vi "Scripting_Server_loop.vi"(4 "error in (no error)":errorcluster, 6 "queue in":refnum<queue>, 7 "TCP Connection ID":refnum<k5>) -> (0 "error out":errorcluster, 3 "Shutdown?":bool)   [LabVIEW 2015]
uses:
  Users/Sherman/Desktop/BETA_GSCS/Systems/SystemUtil/Command.ctl
  Utils/ChangeConfig.ctl
  Utils/ChangeSI.ctl
  Utils/ChangeTCS.ctl
  Users/Sherman/Desktop/BETA_GSCS/Systems/Slit/slitactions.ctl
  TCPServer/TCP_Global.vi
panel:
  out "Focus Done":bool
  out "Focus Commanded":bool
  out "Camset Done":bool
  out "Setup Done":bool
  out "Setup Commanded":bool
  out "Config Server":bool
  out "SI Server":bool
  out "TCS Server":bool
  out "Exposure Active?":bool
  out "Command History":string
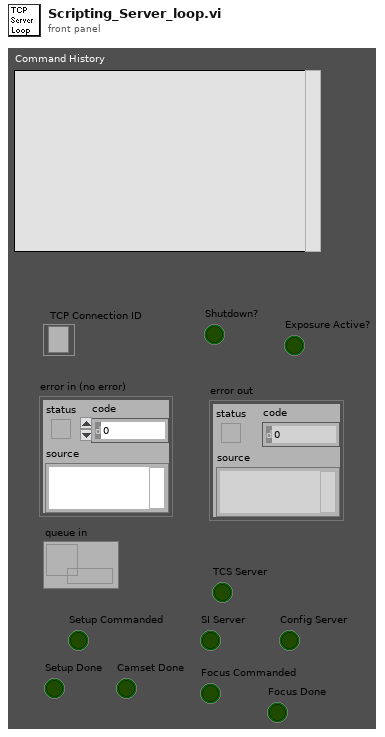
[diagram p1: front panel]
types:
  T1 = typedef "ChangeTCS.ctl" = cluster{"Command":string, "TCS":cluster{"Comp Mirror":bool, "RA":string, "DEC":string, "Epoch":string}}
  T2 = typedef "ChangeSI.ctl" = cluster{"Command":string, "SI camera info":cluster{"Observer Name":string, "object name":string, "File name base":string, "Camera Color":string, "Exp type tab":enum16{"Object", "Flat", "Comp", "Dark", "Zero", "Focus"}, "Number of Exp":i32, "Exp time":i32, "CCD Readout Speed":u8, "CCD ROI Mode":u16, "Hg(Ar)":bool, "Cu":bool, "Ne":bool, "Bulb":bool, "Ar":bool, "Quartz":bool, "Quartz Percent":i32, "Fe":bool, "Notes":string, "Target Number":string, "DomePercent":i32, "Dome":bool, "Start":dbl, "Delta":dbl, "Steps":dbl, "Custom Roi":cluster{i32, i32, i32, i32, i32, i32}}}
  T3 = typedef "ChangeConfig.ctl" = cluster{"Command":string, "Configuration":cluster{"Primary Filter":string, "Secondary Filter":string, "Slit Mask":string, "Grating":string, "CS Target":dbl, "GS Target":dbl, "Coll Focus":i32, "Camera Focus":i32, "use Flexure Comp?":bool, "WavMode":string, "Slit Toggle":string}}
  T4 = typedef "Command.ctl" = cluster{"Command":string, "Parameter":string}
  T5 = typedef "slitactions.ctl" = enum16{"Launch", "INIT_CTL", "Restart", "Show", "Hide", "Home", "Move", "Rotate Only", "Shutdown"}
  T6 = typedef "ThreadStates.ctl" = enum16{"Waiting", "Scripting", "Uninitialized", "Error"}
  T7 = cluster{"GT Thread state":T6, "Slit Thread State":T6, "F1 Thread State":T6, "F2 Thread State":T6, "Coll Thread State":T6, "CF Thread State":T6, "Wavelength Thread State":T6}
  T8 = cluster{"Grating Name":string, "Slit Name":string, "Primary Filter Name":string, "Secondary Filter name":string, "Coll Position":i32, "Camera Focus":i32, "Camera Angle":dbl, "Grating Angle":dbl, "Coll Temp":dbl, "CF Temp\n":dbl, "Camera Target":dbl, "Grating Target":dbl, "WAVMODE":string, "Slit Hidden??":bool}
  T9 = cluster{"String":string, "String":string, "String":string, "String":string, "String":string, "String":string}
  T10 = cluster{"String":dbl, "String":dbl, "String":dbl, "String":dbl, "String":dbl, "String":dbl}
  T11 = cluster{"String":string, "String":string, "String":string, "String":string, "String":string, "String":string, "String":string, "String":string}
  T12 = cluster{"String":bool, "String":bool, "String":bool, "String":bool, "String":bool, "String":bool, "String":bool, "String":bool}
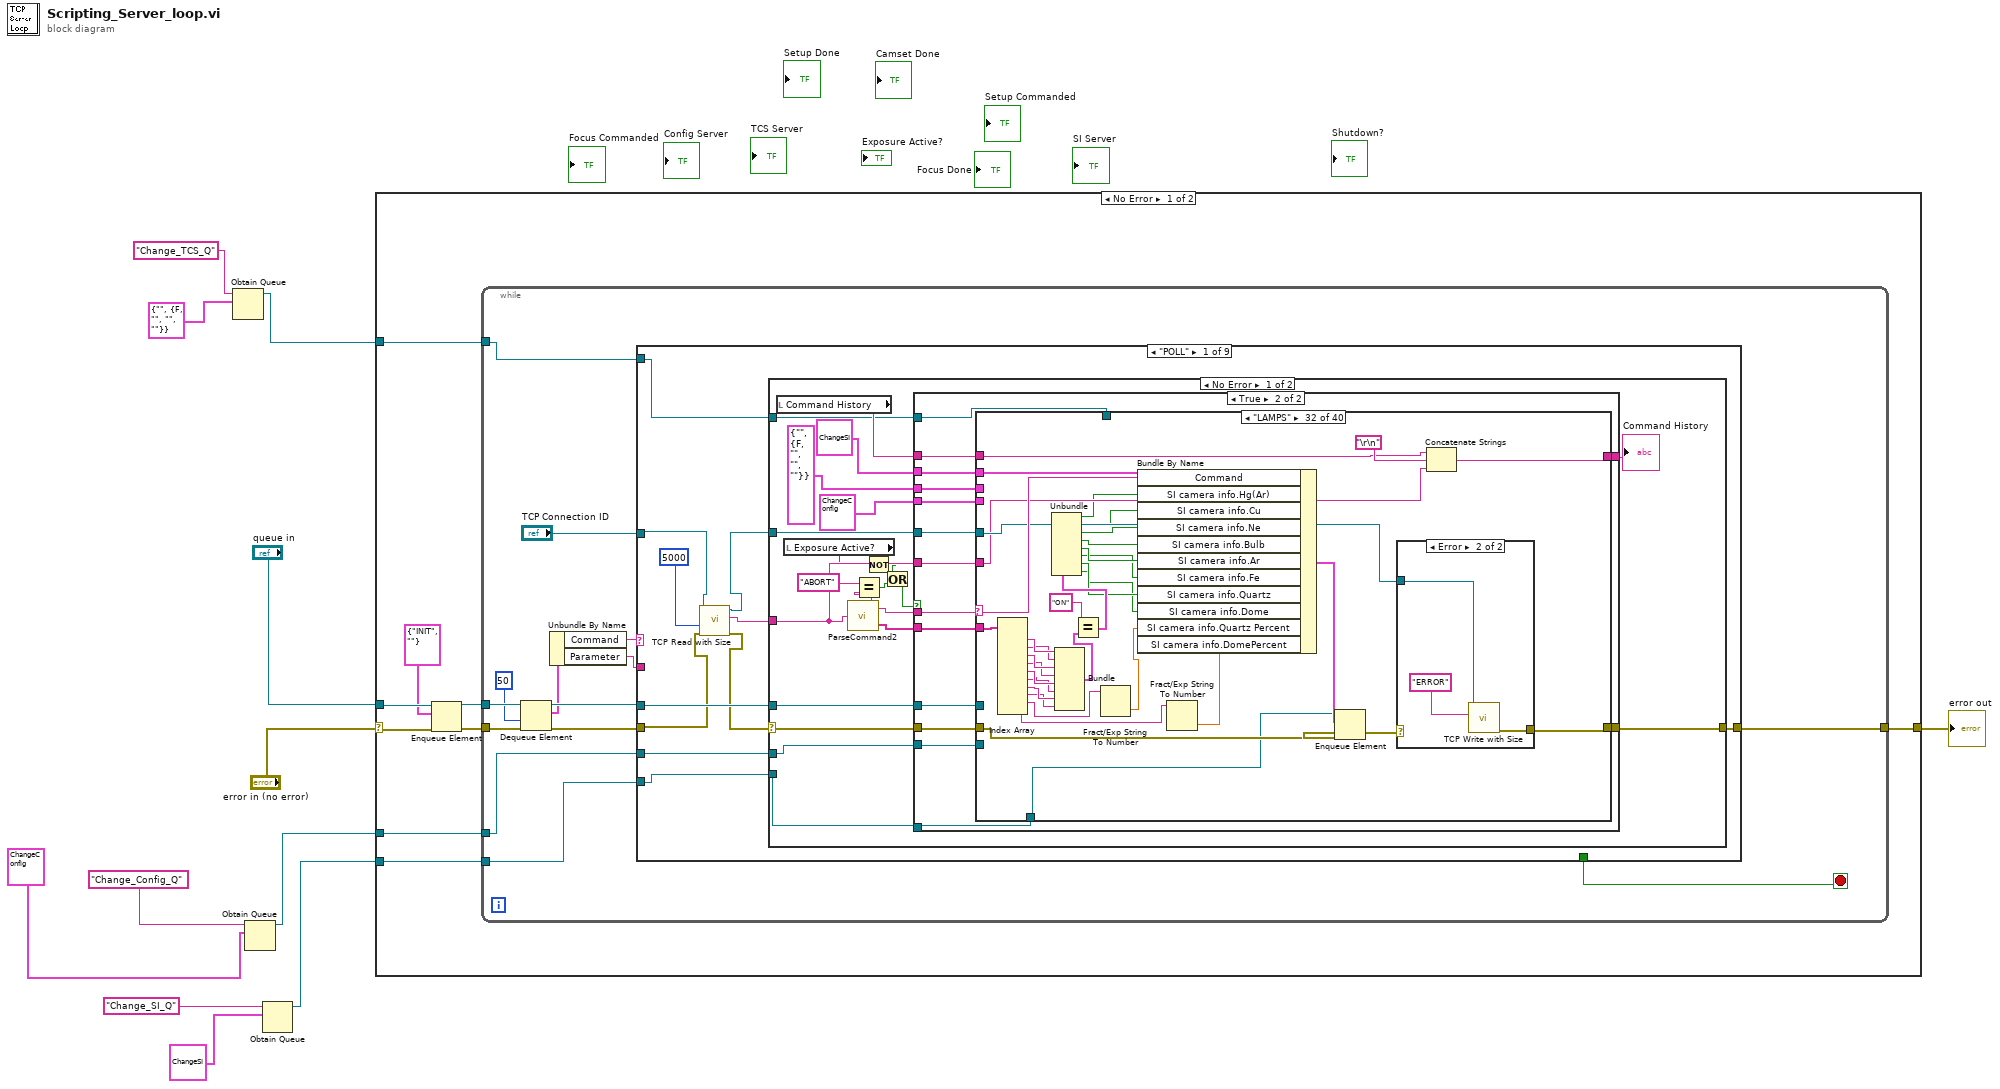
[diagram p0: block diagram]
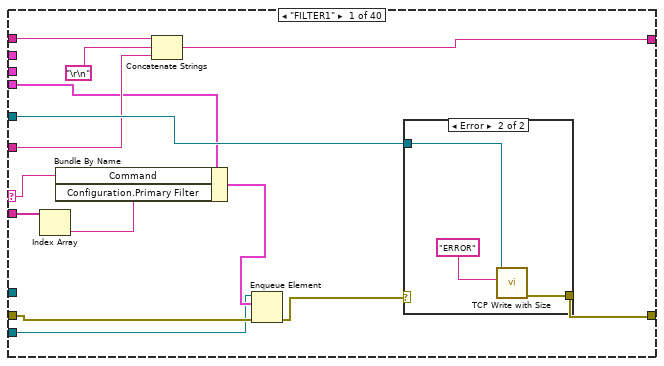
[diagram p3: hidden frame]
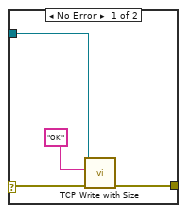
[diagram p4: hidden frame]
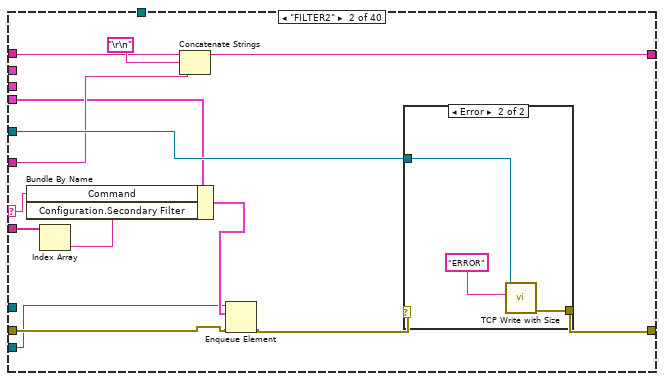
[diagram p5: hidden frame]
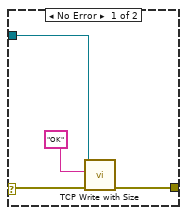
[diagram p6: hidden frame]
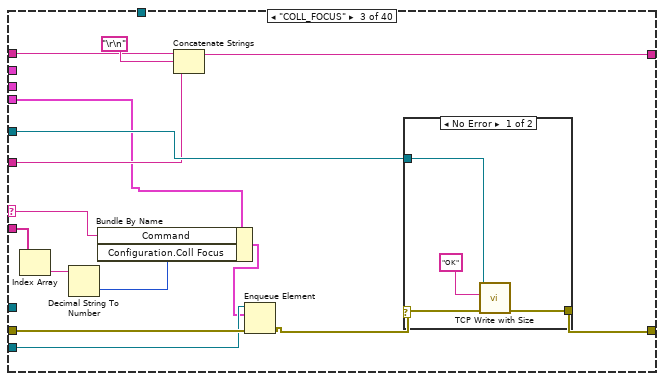
[diagram p7: hidden frame]
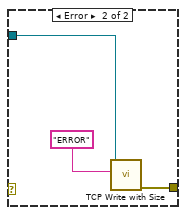
[diagram p8: hidden frame]
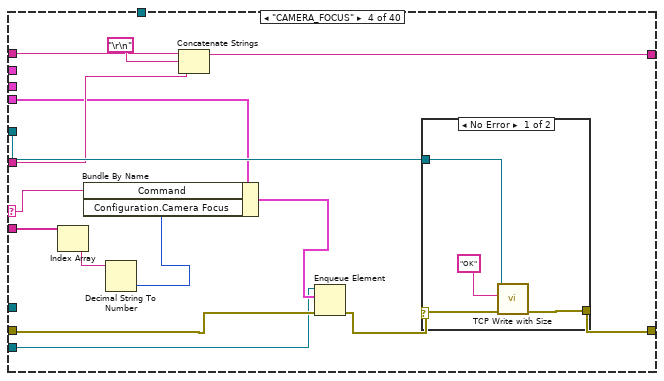
[diagram p9: hidden frame]
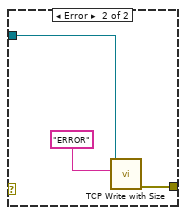
[diagram p10: hidden frame]
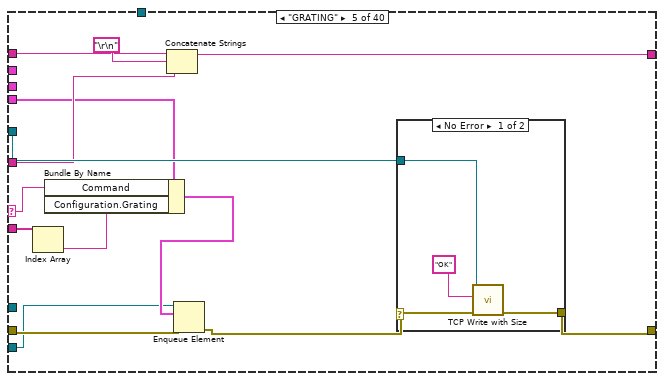
[diagram p11: hidden frame]
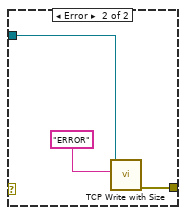
[diagram p12: hidden frame]
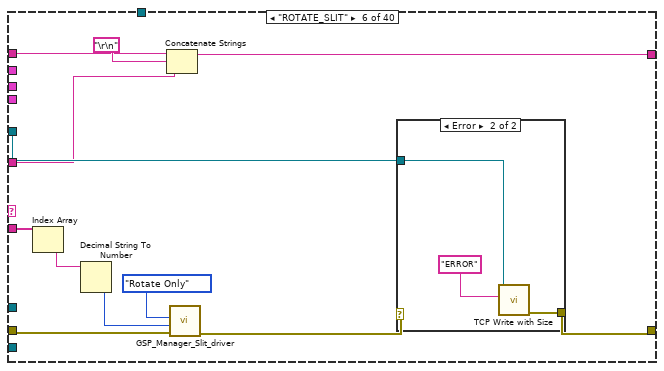
[diagram p13: hidden frame]
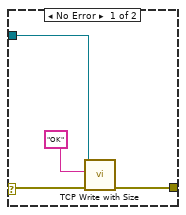
[diagram p14: hidden frame]
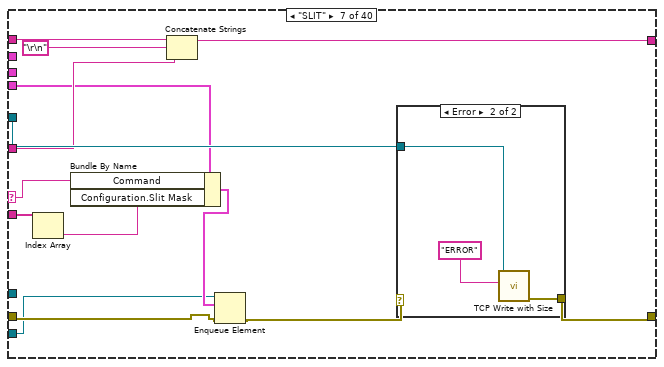
[diagram p15: hidden frame]
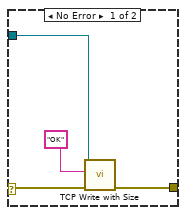
[diagram p16: hidden frame]
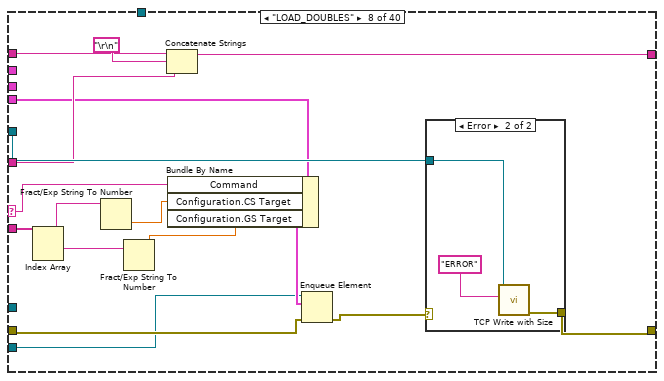
[diagram p17: hidden frame]
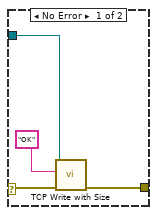
[diagram p18: hidden frame]
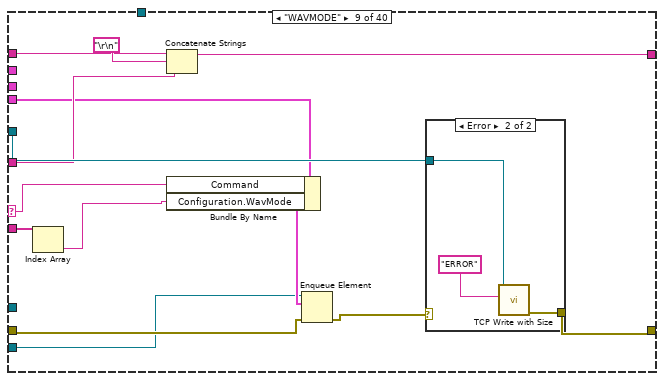
[diagram p19: hidden frame]
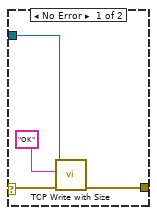
[diagram p20: hidden frame]
diagram:
  n1 = Obtain Queue(name (unnamed)="Change_TCS_Q", element data type=T1 {"Command"="", "TCS"={"Comp Mirror"=FALSE, "RA"="", "DEC"="", "Epoch"=""}} ("Cluster")) -> (queue out=w2:refnum<queue>)  [unwired: 3 in, 2 out]
  n2 = Obtain Queue(name (unnamed)="Change_Config_Q", element data type=T3 {"Command"="", "Configuration"={"Primary Filter"="", "Secondary Filter"="", "Slit Mask"="", "Grating"="", "CS Target"=0.0, "GS Target"=0.0, "Coll Focus"=0, "Camera Focus"=0, "use Flexure Comp?"=FALSE, "WavMode"="", "Slit Toggle"=""}} ("Cluster")) -> (queue out=w8:refnum<queue>)  [unwired: 3 in, 2 out]
  n3 = Obtain Queue(name (unnamed)="Change_SI_Q", element data type=T2 {"Command"="", "SI camera info"={"Observer Name"="", "object name"="", "File name base"="", "Camera Color"="Red", "Exp type tab"=enum."Object", "Number of Exp"=0, "Exp time"=0, "CCD Readout Speed"=5, "CCD ROI Mode"=10, "Hg(Ar)"=FALSE, "Cu"=FALSE, "Ne"=FALSE, "Bulb"=FALSE, "Ar"=FALSE, "Quartz"=FALSE, "Quartz Percent"=0, "Fe"=FALSE, "Notes"="", "Target Number"="", "DomePercent"=0, "Dome"=FALSE, "Start"=0.0, "Delta"=0.0, "Steps"=0.0, "Custom Roi"={0, 4096, 1, 0, 4096, 1}}} ("Cluster")) -> (queue out=w5:refnum<queue>)  [unwired: 3 in, 2 out]
  n4 = case shown="No Error" "error in (no error)" {
    selector: "error in (no error)" -> [w17 w1141]
    tunnel: [w21 w1141] -> w11
    tunnel: "queue in" -> [w18 _]
    tunnel: w8 -> [w15 _]
    tunnel: w5 -> [w14 _]
    tunnel: w2 -> [w13 _]
    frame No Error {
      n5 = Enqueue Element(queue=w18, element=T4 {"Command"="INIT", "Parameter"=""}, error in (no error)=w17) -> (queue out=w20:refnum<queue>, error out=w19:errorcluster)  [unwired: 1 in, 1 out]
      n6 = while {
        tunnel: w20 -> [w35]
        tunnel: [w31] -> w21
        tunnel: w19 -> [w30]
        tunnel: w15 -> [w26]
        tunnel: w14 -> [w25]
        tunnel: w13 -> [w23]
        stop <- w22 stop-if-true
        n7 = Dequeue Element(queue=w35, timeout in ms (-1)=50, error in (no error)=w30) -> (queue out=w33:refnum<queue>, element=w29:T4, error out=w34:errorcluster)  [unwired: 1 out]
        n8 = Unbundle By Name(w29) -> ("Command"=w28:string, "Parameter"=w24:string)
        n9 = case shown="\"POLL\"" w28 {
          tunnel: w33 -> [w45 _ _ _ w1061 _ _ _ _]
          tunnel: w34 -> [w40 w985 w1031 w1056 w1062 w1096 w1101 w1106 w1129]
          tunnel: "TCP Connection ID" -> [w42 w992 w1032 w1057 w1058 _ _ w1105 _]
          tunnel: [w46 w991 w1030 w1055 w1060 w1096 w1101 w1106 w1126] -> w31
          tunnel: [_ _ _ _ _ _ _ TRUE _] -> w22
          tunnel: w26 -> [w44 _ _ _ _ _ _ _ _]
          tunnel: w25 -> [w43 _ _ _ _ _ _ _ _]
          tunnel: w24 -> [_ w986 w1035 w1053 _ w1095 w1100 _ _]
          tunnel: w23 -> [w36 _ _ _ _ _ _ _ _]
          frame "POLL" {
            n10 = call "TCP Read with Size.vi"("error in (no error)"=w40, "timeout ms (25000)"=5000, "connection ID"=w42) -> ("error out"=w39:errorcluster, "data out"=w38:string, "connection ID out"=w37:refnum<k5>)  [unwired: 6 in]
            n11 = case shown="No Error" w39 {
              selector: w39 -> [w64 w980]
              tunnel: w38 -> [w56 _]
              tunnel: w37 -> [w66 _]
              tunnel: [w63 w979] -> w46
              tunnel: w45 -> [w65 _]
              tunnel: w44 -> [w60 _]
              tunnel: w43 -> [w59 _]
              tunnel: w36 -> [w54 _]
              frame No Error {
                n12 = local read "Command History"() -> (w62:string)
                n13 = local read "Exposure Active?"() -> (w50:bool)
                n14 = call "ParseCommand2.vi"("Command string"=w56) -> ("Command"=w51:string, "Parameters"=w55:string[])
                n15 = Equal?(x="ABORT", y=w51) -> (x = y?=w49:bool)
                n16 = Not(x=w50) -> (.not. x?=w48:bool)
                n17 = Or(x=w48, y=w49) -> (x .or. y?=w47:bool)
                n18 = case shown="True" w47 {
                  tunnel: w66 -> [_ w83]
                  tunnel: w65 -> [_ w82]
                  tunnel: w64 -> [w68 w81]
                  tunnel: [w68 w80] -> w63
                  tunnel: w62 -> [w67 w79]
                  tunnel: [w67 w78] -> w61
                  tunnel: w60 -> [_ w77]
                  tunnel: w59 -> [_ w76]
                  tunnel: T3 {"Command"="", "Configuration"={"Primary Filter"="", "Secondary Filter"="", "Slit Mask"="", "Grating"="", "CS Target"=0.0, "GS Target"=0.0, "Coll Focus"=0, "Camera Focus"=0, "use Flexure Comp?"=FALSE, "WavMode"="", "Slit Toggle"=""}} ("Cluster") -> [_ w75]
                  tunnel: T2 {"Command"="", "SI camera info"={"Observer Name"="", "object name"="", "File name base"="Red", "Camera Color"="", "Exp type tab"=enum."Object", "Number of Exp"=0, "Exp time"=0, "CCD Readout Speed"=5, "CCD ROI Mode"=10, "Hg(Ar)"=FALSE, "Cu"=FALSE, "Ne"=FALSE, "Bulb"=FALSE, "Ar"=FALSE, "Quartz"=FALSE, "Quartz Percent"=0, "Fe"=FALSE, "Notes"="", "Target Number"="", "DomePercent"=0, "Dome"=FALSE, "Start"=0.0, "Delta"=0.0, "Steps"=0.0, "Custom Roi"={0, 4096, 1, 0, 4096, 1}}} ("SI camera info") -> [_ w74]
                  tunnel: w56 -> [_ w73]
                  tunnel: w51 -> [_ w72]
                  tunnel: w55 -> [_ w71]
                  tunnel: w54 -> [_ w70]
                  tunnel: T1 {"Command"="", "TCS"={"Comp Mirror"=FALSE, "RA"="", "DEC"="", "Epoch"=""}} ("Cluster") -> [_ w69]
                  frame False {
                    # "do not accept commands other than abort when exposure is active"
                    # "exposure is active and command is not abort"
                  }
                  frame True {
                    n19 = case shown="\"LAMPS\"" w72 {
                      selector: w72 -> [w86 w107 w127 w150 w172 _ w212 w234 w258 w279 w304 _ _ _ w350 w379 w401 w425 w447 w476 w498 w519 w540 w561 w585 w603 w627 w648 w673 w697 w720 w765 w803 w831 w875 w892 w910 _ w947 _]
                      tunnel: w83 -> [w96 w117 w139 w161 w183 w199 w223 w246 w268 w289 w305 w322 w334 w345 w360 w380 w402 w420 w448 w472 w499 w520 w541 w562 w581 w601 w628 w647 w674 w696 w719 w764 w806 w832 w876 w890 w908 w934 w954 w967]
                      tunnel: w71 -> [w97 w118 w140 w159 w182 w197 w222 w245 w267 w288 w303 _ _ _ w357 w378 w400 w424 w446 w475 w497 w518 w539 _ w584 w604 w626 w649 w672 w698 w721 w766 w804 w824 w871 _ _ w925 w949 _]
                      tunnel: w82 -> [_ _ _ _ _ _ _ _ _ _ _ _ _ _ _ _ _ _ _ _ _ _ _ _ _ _ _ _ _ _ _ _ _ _ _ _ _ _ _ _]
                      tunnel: w81 -> [w89 w110 w132 w153 w175 w198 w215 w236 w260 w281 w298 w320 w335 w346 w361 w377 w399 w423 w445 w474 w494 w515 w537 w560 w582 w605 w625 w650 w671 w699 w723 w768 w801 w830 w873 _ _ _ _ w965]
                      tunnel: [w95 w116 w138 w160 w181 w196 w221 w244 w266 w287 w297 w323 w336 w347 w358 w376 w398 w419 w443 w459 w493 w514 w535 w558 w580 w596 w623 w652 w669 w688 w717 w762 w807 w833 w878 w888 w906 w933 w953 w966] -> w80
                      tunnel: w79 -> [w93 w114 w136 w157 w179 w194 w219 w242 w264 w285 w309 w324 w332 w343 w352 w372 w395 w417 w441 w470 w491 w511 w533 w554 w575 w599 w621 w644 w667 w691 w715 w760 w786 w828 w859 w897 w915 w937 w957 w970]
                      tunnel: w73 -> [w92 w112 w134 w155 w177 w192 w217 w240 w262 w283 w306 _ _ _ w349 w371 w393 w415 w440 w469 w490 w510 w532 w553 w574 w598 w620 w643 w666 w690 w714 w759 w785 w827 w858 w896 w914 w936 w956 w969]
                      tunnel: [w94 w113 w135 w156 w178 w193 w218 w241 w263 w284 w308 w324 w332 w343 w351 w373 w394 w416 w439 w468 w489 w512 w531 w552 w573 w597 w619 w642 w665 w689 w713 w758 w784 w826 w860 w895 w913 w935 w955 w968] -> w78
                      tunnel: w77 -> [w84 w105 w131 w148 w170 _ w210 w231 w256 w277 w299 _ _ _ _ _ _ _ _ _ _ _ _ _ _ _ _ _ _ _ _ _ w802 _ _ _ _ _ _ _]
                      tunnel: w76 -> [_ _ _ _ _ _ _ _ _ _ _ _ _ _ w354 w375 w397 w422 w444 w473 w495 w516 w536 w559 w583 w606 w624 w651 w670 w700 w722 w767 _ w819 w874 w891 w909 _ _ _]
                      tunnel: w75 -> [w87 w108 w126 w151 w173 _ w213 w233 w257 w278 w307 _ _ _ _ _ _ _ _ _ _ _ _ _ _ _ _ _ _ _ _ _ w805 _ _ _ _ _ _ _]
                      tunnel: w74 -> [_ _ _ _ _ _ _ _ _ _ _ _ _ _ w362 w381 w403 w421 w449 w477 w500 w521 w542 w563 w586 w602 w629 w646 w675 w695 w718 w763 _ w825 w877 w889 w907 _ _ _]
                      tunnel: w70 -> [_ _ _ _ _ _ _ _ _ _ _ _ _ _ _ _ _ _ _ _ _ _ _ _ _ _ _ _ _ _ _ _ _ _ _ _ _ w932 w952 _]
                      tunnel: w69 -> [_ _ _ _ _ _ _ _ _ _ _ _ _ _ _ _ _ _ _ _ _ _ _ _ _ _ _ _ _ _ _ _ _ _ _ _ _ w931 w951 _]
                      frame "FILTER1" {
                        n20 = Index Array(array=w97) -> (element=w85:string)  [unwired: 1 in]
                        n21 = Bundle By Name(cluster=w87, "Command"=w86, "Configuration.Primary Filter"=w85) -> (w90:T3)
                        n22 = Concatenate Strings(w93, "\r\n", w92) -> (w94:string)
                        n23 = Enqueue Element(queue=w84, element=w90, error in (no error)=w89) -> (error out=w88:errorcluster)  [unwired: 1 in, 2 out]
                        n24 = case shown="Error" w88 {
                          selector: w88 -> [w98 _]
                          tunnel: w96 -> [w100 w102]
                          tunnel: [w99 w103] -> w95
                          frame No Error {
                            n25 = call "TCP Write with Size.vi"("error in (no error)"=w98, "data in"="OK", "connection ID"=w100) -> ("error out"=w99:errorcluster)  [unwired: 6 in, 2 out]
                          }
                          frame Error {
                            n26 = call "TCP Write with Size.vi"("data in"="ERROR", "connection ID"=w102) -> ("error out"=w103:errorcluster)  [unwired: 7 in, 2 out]
                          }
                        }
                      }
                      frame "FILTER2" {
                        n27 = Index Array(array=w118) -> (element=w106:string)  [unwired: 1 in]
                        n28 = Bundle By Name(cluster=w108, "Command"=w107, "Configuration.Secondary Filter"=w106) -> (w111:T3)
                        n29 = Concatenate Strings(w114, "\r\n", w112) -> (w113:string)
                        n30 = Enqueue Element(queue=w105, element=w111, error in (no error)=w110) -> (error out=w109:errorcluster)  [unwired: 1 in, 2 out]
                        n31 = case shown="Error" w109 {
                          selector: w109 -> [w119 _]
                          tunnel: w117 -> [w121 w124]
                          tunnel: [w120 w123] -> w116
                          frame No Error {
                            n32 = call "TCP Write with Size.vi"("error in (no error)"=w119, "data in"="OK", "connection ID"=w121) -> ("error out"=w120:errorcluster)  [unwired: 6 in, 2 out]
                          }
                          frame Error {
                            n33 = call "TCP Write with Size.vi"("data in"="ERROR", "connection ID"=w124) -> ("error out"=w123:errorcluster)  [unwired: 7 in, 2 out]
                          }
                        }
                      }
                      frame "COLL_FOCUS" {
                        n34 = Index Array(array=w140) -> (element=w129:string)  [unwired: 1 in]
                        n35 = Decimal String To Number(string=w129) -> (number=w130:i32)  [unwired: 2 in, 1 out]
                        n36 = Bundle By Name(cluster=w126, "Command"=w127, "Configuration.Coll Focus"=w130) -> (w128:T3)
                        n37 = Concatenate Strings(w136, "\r\n", w134) -> (w135:string)
                        n38 = Enqueue Element(queue=w131, element=w128, error in (no error)=w132) -> (error out=w133:errorcluster)  [unwired: 1 in, 2 out]
                        n39 = case shown="No Error" w133 {
                          selector: w133 -> [w141 _]
                          tunnel: w139 -> [w143 w146]
                          tunnel: [w142 w145] -> w138
                          frame No Error {
                            n40 = call "TCP Write with Size.vi"("error in (no error)"=w141, "data in"="OK", "connection ID"=w143) -> ("error out"=w142:errorcluster)  [unwired: 6 in, 2 out]
                          }
                          frame Error {
                            n41 = call "TCP Write with Size.vi"("data in"="ERROR", "connection ID"=w146) -> ("error out"=w145:errorcluster)  [unwired: 7 in, 2 out]
                          }
                        }
                      }
                      frame "CAMERA_FOCUS" {
                        n42 = Index Array(array=w159) -> (element=w162:string)  [unwired: 1 in]
                        n43 = Decimal String To Number(string=w162) -> (number=w152:i32)  [unwired: 2 in, 1 out]
                        n44 = Bundle By Name(cluster=w151, "Command"=w150, "Configuration.Camera Focus"=w152) -> (w154:T3)
                        n45 = Concatenate Strings(w157, "\r\n", w155) -> (w156:string)
                        n46 = Enqueue Element(queue=w148, element=w154, error in (no error)=w153) -> (error out=w149:errorcluster)  [unwired: 1 in, 2 out]
                        n47 = case shown="No Error" w149 {
                          selector: w149 -> [w163 _]
                          tunnel: w161 -> [w165 w168]
                          tunnel: [w164 w167] -> w160
                          frame No Error {
                            n48 = call "TCP Write with Size.vi"("error in (no error)"=w163, "data in"="OK", "connection ID"=w165) -> ("error out"=w164:errorcluster)  [unwired: 6 in, 2 out]
                          }
                          frame Error {
                            n49 = call "TCP Write with Size.vi"("data in"="ERROR", "connection ID"=w168) -> ("error out"=w167:errorcluster)  [unwired: 7 in, 2 out]
                          }
                        }
                      }
                      frame "GRATING" {
                        n50 = Index Array(array=w182) -> (element=w171:string)  [unwired: 1 in]
                        n51 = Bundle By Name(cluster=w173, "Command"=w172, "Configuration.Grating"=w171) -> (w176:T3)
                        n52 = Concatenate Strings(w179, "\r\n", w177) -> (w178:string)
                        n53 = Enqueue Element(queue=w170, element=w176, error in (no error)=w175) -> (error out=w174:errorcluster)  [unwired: 1 in, 2 out]
                        n54 = case shown="No Error" w174 {
                          selector: w174 -> [w184 _]
                          tunnel: w183 -> [w186 w189]
                          tunnel: [w185 w188] -> w181
                          frame No Error {
                            n55 = call "TCP Write with Size.vi"("error in (no error)"=w184, "data in"="OK", "connection ID"=w186) -> ("error out"=w185:errorcluster)  [unwired: 6 in, 2 out]
                          }
                          frame Error {
                            n56 = call "TCP Write with Size.vi"("data in"="ERROR", "connection ID"=w189) -> ("error out"=w188:errorcluster)  [unwired: 7 in, 2 out]
                          }
                        }
                      }
                      frame "ROTATE_SLIT" {
                        n57 = Index Array(array=w197) -> (element=w202:string)  [unwired: 1 in]
                        n58 = Decimal String To Number(string=w202) -> (number=w201:i32)  [unwired: 2 in, 1 out]
                        n59 = Concatenate Strings(w194, "\r\n", w192) -> (w193:string)
                        n60 = call "GSP_Manager_Slit_driver.vi"("error in (no error)"=w198, "Slit # (Move/Rotate Only)"=w201, "Action"=slitactions."Rotate Only") -> ("error out"=w200:errorcluster)  [unwired: 3 in, 1 out]
                        n61 = case shown="Error" w200 {
                          selector: w200 -> [w203 _]
                          tunnel: w199 -> [w205 w208]
                          tunnel: [w204 w207] -> w196
                          frame No Error {
                            n62 = call "TCP Write with Size.vi"("error in (no error)"=w203, "data in"="OK", "connection ID"=w205) -> ("error out"=w204:errorcluster)  [unwired: 6 in, 2 out]
                          }
                          frame Error {
                            n63 = call "TCP Write with Size.vi"("data in"="ERROR", "connection ID"=w208) -> ("error out"=w207:errorcluster)  [unwired: 7 in, 2 out]
                          }
                        }
                      }
                      frame "SLIT" {
                        n64 = Index Array(array=w222) -> (element=w211:string)  [unwired: 1 in]
                        n65 = Bundle By Name(cluster=w213, "Command"=w212, "Configuration.Slit Mask"=w211) -> (w216:T3)
                        n66 = Concatenate Strings(w219, "\r\n", w217) -> (w218:string)
                        n67 = Enqueue Element(queue=w210, element=w216, error in (no error)=w215) -> (error out=w214:errorcluster)  [unwired: 1 in, 2 out]
                        n68 = case shown="Error" w214 {
                          selector: w214 -> [w224 _]
                          tunnel: w223 -> [w226 w229]
                          tunnel: [w225 w228] -> w221
                          frame No Error {
                            n69 = call "TCP Write with Size.vi"("error in (no error)"=w224, "data in"="OK", "connection ID"=w226) -> ("error out"=w225:errorcluster)  [unwired: 6 in, 2 out]
                          }
                          frame Error {
                            n70 = call "TCP Write with Size.vi"("data in"="ERROR", "connection ID"=w229) -> ("error out"=w228:errorcluster)  [unwired: 7 in, 2 out]
                          }
                        }
                      }
                      frame "LOAD_DOUBLES" {
                        n71 = Index Array(array=w245) -> (element #1=w247:string, element #2=w239:string)  [unwired: 2 in]
                        n72 = Fract/Exp String To Number(string=w247) -> (number=w232:dbl)  [unwired: 3 in, 1 out]
                        n73 = Fract/Exp String To Number(string=w239) -> (number=w237:dbl)  [unwired: 3 in, 1 out]
                        n74 = Concatenate Strings(w242, "\r\n", w240) -> (w241:string)
                        n75 = Bundle By Name(cluster=w233, "Command"=w234, "Configuration.CS Target"=w232, "Configuration.GS Target"=w237) -> (w238:T3)
                        n76 = Enqueue Element(queue=w231, element=w238, error in (no error)=w236) -> (error out=w235:errorcluster)  [unwired: 1 in, 2 out]
                        n77 = case shown="Error" w235 {
                          selector: w235 -> [w248 _]
                          tunnel: w246 -> [w250 w253]
                          tunnel: [w249 w252] -> w244
                          frame No Error {
                            n78 = call "TCP Write with Size.vi"("error in (no error)"=w248, "data in"="OK", "connection ID"=w250) -> ("error out"=w249:errorcluster)  [unwired: 6 in, 2 out]
                          }
                          frame Error {
                            n79 = call "TCP Write with Size.vi"("data in"="ERROR", "connection ID"=w253) -> ("error out"=w252:errorcluster)  [unwired: 7 in, 2 out]
                          }
                        }
                      }
                      frame "WAVMODE" {
                        n80 = Index Array(array=w267) -> (element=w255:string)  [unwired: 1 in]
                        n81 = Concatenate Strings(w264, "\r\n", w262) -> (w263:string)
                        n82 = Bundle By Name(cluster=w257, "Command"=w258, "Configuration.WavMode"=w255) -> (w261:T3)
                        n83 = Enqueue Element(queue=w256, element=w261, error in (no error)=w260) -> (error out=w259:errorcluster)  [unwired: 1 in, 2 out]
                        n84 = case shown="Error" w259 {
                          selector: w259 -> [w269 _]
                          tunnel: w268 -> [w271 w274]
                          tunnel: [w270 w273] -> w266
                          frame No Error {
                            n85 = call "TCP Write with Size.vi"("error in (no error)"=w269, "data in"="OK", "connection ID"=w271) -> ("error out"=w270:errorcluster)  [unwired: 6 in, 2 out]
                          }
                          frame Error {
                            n86 = call "TCP Write with Size.vi"("data in"="ERROR", "connection ID"=w274) -> ("error out"=w273:errorcluster)  [unwired: 7 in, 2 out]
                          }
                        }
                      }
                      frame "SLIT_TOG" {
                        n87 = Index Array(array=w288) -> (element=w276:string)  [unwired: 1 in]
                        n88 = Bundle By Name(cluster=w278, "Command"=w279, "Configuration.Slit Toggle"=w276) -> (w282:T3)
                        n89 = Concatenate Strings(w285, "\r\n", w283) -> (w284:string)
                        n90 = Enqueue Element(queue=w277, element=w282, error in (no error)=w281) -> (error out=w280:errorcluster)  [unwired: 1 in, 2 out]
                        n91 = case shown="Error" w280 {
                          selector: w280 -> [w290 _]
                          tunnel: w289 -> [w292 w295]
                          tunnel: [w291 w294] -> w287
                          frame No Error {
                            n92 = call "TCP Write with Size.vi"("error in (no error)"=w290, "data in"="OK", "connection ID"=w292) -> ("error out"=w291:errorcluster)  [unwired: 6 in, 2 out]
                          }
                          frame Error {
                            n93 = call "TCP Write with Size.vi"("data in"="ERROR", "connection ID"=w295) -> ("error out"=w294:errorcluster)  [unwired: 7 in, 2 out]
                          }
                        }
                      }
                      frame "FLEXURE" {
                        n94 = Index Array(array=w303) -> (element=w301:string)  [unwired: 1 in]
                        n95 = Equal?(x="ON", y=w301) -> (x = y?=w300:bool)
                        n96 = Bundle By Name(cluster=w307, "Command"=w304, "Configuration.use Flexure Comp?"=w300) -> (w311:T3)
                        n97 = Concatenate Strings(w309, "\r\n", w306) -> (w308:string)
                        n98 = Enqueue Element(queue=w299, element=w311, error in (no error)=w298) -> (error out=w310:errorcluster)  [unwired: 1 in, 2 out]
                        n99 = case shown="No Error" w310 {
                          selector: w310 -> [w313 _]
                          tunnel: w305 -> [w315 w318]
                          tunnel: [w314 w317] -> w297
                          frame No Error {
                            n100 = call "TCP Write with Size.vi"("error in (no error)"=w313, "data in"="OK", "connection ID"=w315) -> ("error out"=w314:errorcluster)  [unwired: 6 in, 2 out]
                          }
                          frame Error {
                            n101 = call "TCP Write with Size.vi"("data in"="ERROR", "connection ID"=w318) -> ("error out"=w317:errorcluster)  [unwired: 7 in, 2 out]
                          }
                        }
                      }
                      frame "QUIT", Default {
                        w321 = TRUE
                        n102 = local write "Shutdown?"(w321) -> ()
                        n103 = global write "TCP_Global.vi" "Shutdown"(w321) -> ()
                        n104 = case shown="Error" w320 {
                          selector: w320 -> [w325 _]
                          tunnel: w322 -> [w327 w330]
                          tunnel: [w326 w329] -> w323
                          frame No Error {
                            n105 = call "TCP Write with Size.vi"("error in (no error)"=w325, "data in"="OK", "connection ID"=w327) -> ("error out"=w326:errorcluster)  [unwired: 6 in, 2 out]
                          }
                          frame Error {
                            n106 = call "TCP Write with Size.vi"("data in"="ERROR", "connection ID"=w330) -> ("error out"=w329:errorcluster)  [unwired: 7 in, 2 out]
                          }
                        }
                      }
                      frame "SYSTEM_STATUS" {
                        n107 = call "GetSystemsStatus.vi"() -> ("Thread States"=w340:T7)  [unwired: 4 in, 3 out]
                        n108 = Cluster To Array(cluster=w340) -> (array=w339:T6[])
                        n109 = Number To Decimal String(number=w339) -> (decimal integer string=w338:string[])  [unwired: 1 in]
                        n110 = call "FormCommand.vi"("Parameters"=w338, "Command"="OK") -> ("Command string"=w333:string)
                        n111 = call "TCP Write with Size.vi"("error in (no error)"=w335, "data in"=w333, "connection ID"=w334) -> ("error out"=w336:errorcluster)  [unwired: 6 in, 2 out]
                      }
                      frame "SYSTEM_POS" {
                        n112 = call "GetSystemInfoNames.vi"() -> ("Pos Info"=w342:T8)  [unwired: 11 in]
                        n113 = call "FormatPositions.vi"("Pos Info"=w342) -> ("Pos strings"=w341:string[])
                        n114 = call "FormCommand.vi"("Parameters"=w341, "Command"="OK") -> ("Command string"=w344:string)
                        n115 = call "TCP Write with Size.vi"("error in (no error)"=w346, "data in"=w344, "connection ID"=w345) -> ("error out"=w347:errorcluster)  [unwired: 6 in, 2 out]
                      }
                      frame "EXP_TIME " {
                        n116 = Index Array(array=w357) -> (element=w356:string)  [unwired: 1 in]
                        n117 = Fract/Exp String To Number(string=w356) -> (number=w355:dbl)  [unwired: 3 in, 1 out]
                        n118 = Bundle By Name(cluster=w362, "Command"=w350, "SI camera info.Exp time"=w355) -> (w363:T2)
                        n119 = Enqueue Element(queue=w354, element=w363, error in (no error)=w361) -> (error out=w359:errorcluster)  [unwired: 1 in, 2 out]
                        n120 = case shown="Error" w359 {
                          selector: w359 -> [w364 _]
                          tunnel: w360 -> [w366 w369]
                          tunnel: [w365 w368] -> w358
                          frame No Error {
                            n121 = call "TCP Write with Size.vi"("error in (no error)"=w364, "data in"="OK", "connection ID"=w366) -> ("error out"=w365:errorcluster)  [unwired: 6 in, 2 out]
                          }
                          frame Error {
                            n122 = call "TCP Write with Size.vi"("data in"="ERROR", "connection ID"=w369) -> ("error out"=w368:errorcluster)  [unwired: 7 in, 2 out]
                          }
                        }
                        n123 = Concatenate Strings(w352, "\r\n", w349) -> (w351:string)
                      }
                      frame "EXPNUM" {
                        n124 = Index Array(array=w378) -> (element=w383:string)  [unwired: 1 in]
                        n125 = Fract/Exp String To Number(string=w383) -> (number=w382:dbl)  [unwired: 3 in, 1 out]
                        n126 = Bundle By Name(cluster=w381, "Command"=w379, "SI camera info.Number of Exp"=w382) -> (w385:T2)
                        n127 = Enqueue Element(queue=w375, element=w385, error in (no error)=w377) -> (error out=w384:errorcluster)  [unwired: 1 in, 2 out]
                        n128 = case shown="No Error" w384 {
                          selector: w384 -> [w386 _]
                          tunnel: w380 -> [w388 w391]
                          tunnel: [w387 w390] -> w376
                          frame No Error {
                            n129 = call "TCP Write with Size.vi"("error in (no error)"=w386, "data in"="OK", "connection ID"=w388) -> ("error out"=w387:errorcluster)  [unwired: 6 in, 2 out]
                          }
                          frame Error {
                            n130 = call "TCP Write with Size.vi"("data in"="ERROR", "connection ID"=w391) -> ("error out"=w390:errorcluster)  [unwired: 7 in, 2 out]
                          }
                        }
                        n131 = Concatenate Strings(w372, "\r\n", w371) -> (w373:string)
                      }
                      frame "ROI" {
                        n132 = Index Array(array=w400) -> (element=w405:string)  [unwired: 1 in]
                        n133 = Fract/Exp String To Number(string=w405) -> (number=w404:dbl)  [unwired: 3 in, 1 out]
                        n134 = Bundle By Name(cluster=w403, "Command"=w401, "SI camera info.CCD ROI Mode"=w404) -> (w407:T2)
                        n135 = Enqueue Element(queue=w397, element=w407, error in (no error)=w399) -> (error out=w406:errorcluster)  [unwired: 1 in, 2 out]
                        n136 = case shown="Error" w406 {
                          selector: w406 -> [w408 _]
                          tunnel: w402 -> [w410 w413]
                          tunnel: [w409 w412] -> w398
                          frame No Error {
                            n137 = call "TCP Write with Size.vi"("error in (no error)"=w408, "data in"="OK", "connection ID"=w410) -> ("error out"=w409:errorcluster)  [unwired: 6 in, 2 out]
                          }
                          frame Error {
                            n138 = call "TCP Write with Size.vi"("data in"="ERROR", "connection ID"=w413) -> ("error out"=w412:errorcluster)  [unwired: 7 in, 2 out]
                          }
                        }
                        n139 = Concatenate Strings(w395, "\r\n", w393) -> (w394:string)
                      }
                      frame "ROSPEED" {
                        n140 = Index Array(array=w424) -> (element=w427:string)  [unwired: 1 in]
                        n141 = Fract/Exp String To Number(string=w427) -> (number=w426:dbl)  [unwired: 3 in, 1 out]
                        n142 = Bundle By Name(cluster=w421, "Command"=w425, "SI camera info.CCD Readout Speed"=w426) -> (w429:T2)
                        n143 = Enqueue Element(queue=w422, element=w429, error in (no error)=w423) -> (error out=w428:errorcluster)  [unwired: 1 in, 2 out]
                        n144 = case shown="Error" w428 {
                          selector: w428 -> [w430 _]
                          tunnel: w420 -> [w432 w435]
                          tunnel: [w431 w434] -> w419
                          frame No Error {
                            n145 = call "TCP Write with Size.vi"("error in (no error)"=w430, "data in"="OK", "connection ID"=w432) -> ("error out"=w431:errorcluster)  [unwired: 6 in, 2 out]
                          }
                          frame Error {
                            n146 = call "TCP Write with Size.vi"("data in"="ERROR", "connection ID"=w435) -> ("error out"=w434:errorcluster)  [unwired: 7 in, 2 out]
                          }
                        }
                        n147 = Concatenate Strings(w417, "\r\n", w415) -> (w416:string)
                      }
                      frame "ROTYPE" {
                        n148 = Index Array(array=w446) -> (element=w438:string)  [unwired: 1 in]
                        n149 = Fract/Exp String To Number(string=w438) -> (number=w437:dbl)  [unwired: 3 in, 1 out]
                        n150 = Bundle By Name(cluster=w449, "Command"=w447, "SI camera info.Exp type tab"=w437) -> (w451:T2)
                        n151 = Enqueue Element(queue=w444, element=w451, error in (no error)=w445) -> (error out=w450:errorcluster)  [unwired: 1 in, 2 out]
                        n152 = Concatenate Strings(w441, "\r\n", w440) -> (w439:string)
                        n153 = case shown="Error" w450 {
                          selector: w450 -> [w452 _]
                          tunnel: w448 -> [w454 w457]
                          tunnel: [w453 w456] -> w443
                          frame No Error {
                            n154 = call "TCP Write with Size.vi"("error in (no error)"=w452, "data in"="OK", "connection ID"=w454) -> ("error out"=w453:errorcluster)  [unwired: 6 in, 2 out]
                          }
                          frame Error {
                            n155 = call "TCP Write with Size.vi"("data in"="ERROR", "connection ID"=w457) -> ("error out"=w456:errorcluster)  [unwired: 7 in, 2 out]
                          }
                        }
                      }
                      frame "CUSTOMROI" {
                        n156 = Index Array(array=w475) -> (element #1=w479:string, element #2=w467:string, element #3=w466:string, element #4=w465:string, element #5=w464:string, element #6=w463:string, element #7=w462:string)  [unwired: 7 in]
                        n157 = Bundle("String"=w467, "String"=w466, "String"=w465, "String"=w464, "String"=w463, "String"=w462) -> (w461:T9)  [unwired: 1 in]
                        n158 = Fract/Exp String To Number(string=w479) -> (number=w478:dbl)  [unwired: 3 in, 1 out]
                        n159 = Fract/Exp String To Number(string=w461) -> (number=w460:T10)  [unwired: 3 in, 1 out]
                        n160 = Bundle By Name(cluster=w477, "Command"=w476, "SI camera info.CCD ROI Mode"=w478, "SI camera info.Custom Roi"=w460) -> (w481:T2)
                        n161 = Enqueue Element(queue=w473, element=w481, error in (no error)=w474) -> (error out=w480:errorcluster)  [unwired: 1 in, 2 out]
                        n162 = Concatenate Strings(w470, "\r\n", w469) -> (w468:string)
                        n163 = case shown="Error" w480 {
                          selector: w480 -> [w482 _]
                          tunnel: w472 -> [w484 w487]
                          tunnel: [w483 w486] -> w459
                          frame No Error {
                            n164 = call "TCP Write with Size.vi"("error in (no error)"=w482, "data in"="OK", "connection ID"=w484) -> ("error out"=w483:errorcluster)  [unwired: 6 in, 2 out]
                          }
                          frame Error {
                            n165 = call "TCP Write with Size.vi"("data in"="ERROR", "connection ID"=w487) -> ("error out"=w486:errorcluster)  [unwired: 7 in, 2 out]
                          }
                        }
                      }
                      frame "FILENAME" {
                        n166 = Index Array(array=w497) -> (element=w496:string)  [unwired: 1 in]
                        n167 = Bundle By Name(cluster=w500, "Command"=w498, "SI camera info.File name base"=w496) -> (w502:T2)
                        n168 = Enqueue Element(queue=w495, element=w502, error in (no error)=w494) -> (error out=w501:errorcluster)  [unwired: 1 in, 2 out]
                        n169 = Concatenate Strings(w491, "\r\n", w490) -> (w489:string)
                        n170 = case shown="Error" w501 {
                          selector: w501 -> [w503 _]
                          tunnel: w499 -> [w505 w508]
                          tunnel: [w504 w507] -> w493
                          frame No Error {
                            n171 = call "TCP Write with Size.vi"("error in (no error)"=w503, "data in"="OK", "connection ID"=w505) -> ("error out"=w504:errorcluster)  [unwired: 6 in, 2 out]
                          }
                          frame Error {
                            n172 = call "TCP Write with Size.vi"("data in"="ERROR", "connection ID"=w508) -> ("error out"=w507:errorcluster)  [unwired: 7 in, 2 out]
                          }
                        }
                      }
                      frame "OBSNAME" {
                        n173 = Index Array(array=w518) -> (element=w517:string)  [unwired: 1 in]
                        n174 = Bundle By Name(cluster=w521, "Command"=w519, "SI camera info.Observer Name"=w517) -> (w523:T2)
                        n175 = Enqueue Element(queue=w516, element=w523, error in (no error)=w515) -> (error out=w522:errorcluster)  [unwired: 1 in, 2 out]
                        n176 = case shown="Error" w522 {
                          selector: w522 -> [w524 _]
                          tunnel: w520 -> [w526 w529]
                          tunnel: [w525 w528] -> w514
                          frame No Error {
                            n177 = call "TCP Write with Size.vi"("error in (no error)"=w524, "data in"="OK", "connection ID"=w526) -> ("error out"=w525:errorcluster)  [unwired: 6 in, 2 out]
                          }
                          frame Error {
                            n178 = call "TCP Write with Size.vi"("data in"="ERROR", "connection ID"=w529) -> ("error out"=w528:errorcluster)  [unwired: 7 in, 2 out]
                          }
                        }
                        n179 = Concatenate Strings(w511, "\r\n", w510) -> (w512:string)
                      }
                      frame "OBJNAME" {
                        n180 = Index Array(array=w539) -> (element=w538:string)  [unwired: 1 in]
                        n181 = Bundle By Name(cluster=w542, "Command"=w540, "SI camera info.Observer Name"=w538) -> (w544:T2)
                        n182 = Enqueue Element(queue=w536, element=w544, error in (no error)=w537) -> (error out=w543:errorcluster)  [unwired: 1 in, 2 out]
                        n183 = case shown="Error" w543 {
                          selector: w543 -> [w545 _]
                          tunnel: w541 -> [w547 w550]
                          tunnel: [w546 w549] -> w535
                          frame No Error {
                            n184 = call "TCP Write with Size.vi"("error in (no error)"=w545, "data in"="OK", "connection ID"=w547) -> ("error out"=w546:errorcluster)  [unwired: 6 in, 2 out]
                          }
                          frame Error {
                            n185 = call "TCP Write with Size.vi"("data in"="ERROR", "connection ID"=w550) -> ("error out"=w549:errorcluster)  [unwired: 7 in, 2 out]
                          }
                        }
                        n186 = Concatenate Strings(w533, "\r\n", w532) -> (w531:string)
                      }
                      frame "NOTES" {
                        n187 = Match Pattern(string=w553, regular expression=" ") -> (after substring=w556:string)  [unwired: 1 in, 3 out]
                        n188 = Bundle By Name(cluster=w563, "Command"=w561, "SI camera info.Notes"=w556) -> (w565:T2)
                        n189 = Enqueue Element(queue=w559, element=w565, error in (no error)=w560) -> (error out=w564:errorcluster)  [unwired: 1 in, 2 out]
                        n190 = case shown="Error" w564 {
                          selector: w564 -> [w566 _]
                          tunnel: w562 -> [w568 w571]
                          tunnel: [w567 w570] -> w558
                          frame No Error {
                            n191 = call "TCP Write with Size.vi"("error in (no error)"=w566, "data in"="OK", "connection ID"=w568) -> ("error out"=w567:errorcluster)  [unwired: 6 in, 2 out]
                          }
                          frame Error {
                            n192 = call "TCP Write with Size.vi"("data in"="ERROR", "connection ID"=w571) -> ("error out"=w570:errorcluster)  [unwired: 7 in, 2 out]
                          }
                        }
                        n193 = Concatenate Strings(w554, "\r\n", w553) -> (w552:string)
                      }
                      frame "Hg(Ar)" {
                        n194 = Index Array(array=w584) -> (element=w578:string)  [unwired: 1 in]
                        n195 = Equal?(x="ON", y=w578) -> (x = y?=w577:bool)
                        n196 = Bundle By Name(cluster=w586, "Command"=w585, "SI camera info.Hg(Ar)"=w577) -> (w588:T2)
                        n197 = Enqueue Element(queue=w583, element=w588, error in (no error)=w582) -> (error out=w587:errorcluster)  [unwired: 1 in, 2 out]
                        n198 = case shown="Error" w587 {
                          selector: w587 -> [w589 _]
                          tunnel: w581 -> [w591 w594]
                          tunnel: [w590 w593] -> w580
                          frame No Error {
                            n199 = call "TCP Write with Size.vi"("error in (no error)"=w589, "data in"="OK", "connection ID"=w591) -> ("error out"=w590:errorcluster)  [unwired: 6 in, 2 out]
                          }
                          frame Error {
                            n200 = call "TCP Write with Size.vi"("data in"="ERROR", "connection ID"=w594) -> ("error out"=w593:errorcluster)  [unwired: 7 in, 2 out]
                          }
                        }
                        n201 = Concatenate Strings(w575, "\r\n", w574) -> (w573:string)
                      }
                      frame "Cu" {
                        n202 = Index Array(array=w604) -> (element=w608:string)  [unwired: 1 in]
                        n203 = Equal?(x="ON", y=w608) -> (x = y?=w607:bool)
                        n204 = Bundle By Name(cluster=w602, "Command"=w603, "SI camera info.Cu"=w607) -> (w611:T2)
                        n205 = Enqueue Element(queue=w606, element=w611, error in (no error)=w605) -> (error out=w610:errorcluster)  [unwired: 1 in, 2 out]
                        n206 = case shown="Error" w610 {
                          selector: w610 -> [w612 _]
                          tunnel: w601 -> [w614 w617]
                          tunnel: [w613 w616] -> w596
                          frame No Error {
                            n207 = call "TCP Write with Size.vi"("error in (no error)"=w612, "data in"="OK", "connection ID"=w614) -> ("error out"=w613:errorcluster)  [unwired: 6 in, 2 out]
                          }
                          frame Error {
                            n208 = call "TCP Write with Size.vi"("data in"="ERROR", "connection ID"=w617) -> ("error out"=w616:errorcluster)  [unwired: 7 in, 2 out]
                          }
                        }
                        n209 = Concatenate Strings(w599, "\r\n", w598) -> (w597:string)
                      }
                      frame "Ne" {
                        n210 = Index Array(array=w626) -> (element=w631:string)  [unwired: 1 in]
                        n211 = Equal?(x="ON", y=w631) -> (x = y?=w630:bool)
                        n212 = Bundle By Name(cluster=w629, "Command"=w627, "SI camera info.Ne"=w630) -> (w634:T2)
                        n213 = Enqueue Element(queue=w624, element=w634, error in (no error)=w625) -> (error out=w633:errorcluster)  [unwired: 1 in, 2 out]
                        n214 = case shown="Error" w633 {
                          selector: w633 -> [w635 _]
                          tunnel: w628 -> [w637 w640]
                          tunnel: [w636 w639] -> w623
                          frame No Error {
                            n215 = call "TCP Write with Size.vi"("error in (no error)"=w635, "data in"="OK", "connection ID"=w637) -> ("error out"=w636:errorcluster)  [unwired: 6 in, 2 out]
                          }
                          frame Error {
                            n216 = call "TCP Write with Size.vi"("data in"="ERROR", "connection ID"=w640) -> ("error out"=w639:errorcluster)  [unwired: 7 in, 2 out]
                          }
                        }
                        n217 = Concatenate Strings(w621, "\r\n", w620) -> (w619:string)
                      }
                      frame "Bulb" {
                        n218 = Index Array(array=w649) -> (element=w654:string)  [unwired: 1 in]
                        n219 = Equal?(x="ON", y=w654) -> (x = y?=w653:bool)
                        n220 = Bundle By Name(cluster=w646, "Command"=w648, "SI camera info.Bulb"=w653) -> (w657:T2)
                        n221 = Enqueue Element(queue=w651, element=w657, error in (no error)=w650) -> (error out=w656:errorcluster)  [unwired: 1 in, 2 out]
                        n222 = Concatenate Strings(w644, "\r\n", w643) -> (w642:string)
                        n223 = case shown="Error" w656 {
                          selector: w656 -> [w658 _]
                          tunnel: w647 -> [w660 w663]
                          tunnel: [w659 w662] -> w652
                          frame No Error {
                            n224 = call "TCP Write with Size.vi"("error in (no error)"=w658, "data in"="OK", "connection ID"=w660) -> ("error out"=w659:errorcluster)  [unwired: 6 in, 2 out]
                          }
                          frame Error {
                            n225 = call "TCP Write with Size.vi"("data in"="ERROR", "connection ID"=w663) -> ("error out"=w662:errorcluster)  [unwired: 7 in, 2 out]
                          }
                        }
                      }
                      frame "Ar" {
                        n226 = Index Array(array=w672) -> (element=w677:string)  [unwired: 1 in]
                        n227 = Equal?(x="ON", y=w677) -> (x = y?=w676:bool)
                        n228 = Bundle By Name(cluster=w675, "Command"=w673, "SI camera info.Ar"=w676) -> (w680:T2)
                        n229 = Enqueue Element(queue=w670, element=w680, error in (no error)=w671) -> (error out=w679:errorcluster)  [unwired: 1 in, 2 out]
                        n230 = case shown="Error" w679 {
                          selector: w679 -> [w681 _]
                          tunnel: w674 -> [w683 w686]
                          tunnel: [w682 w685] -> w669
                          frame No Error {
                            n231 = call "TCP Write with Size.vi"("error in (no error)"=w681, "data in"="OK", "connection ID"=w683) -> ("error out"=w682:errorcluster)  [unwired: 6 in, 2 out]
                          }
                          frame Error {
                            n232 = call "TCP Write with Size.vi"("data in"="ERROR", "connection ID"=w686) -> ("error out"=w685:errorcluster)  [unwired: 7 in, 2 out]
                          }
                        }
                        n233 = Concatenate Strings(w667, "\r\n", w666) -> (w665:string)
                      }
                      frame "Quartz" {
                        n234 = Index Array(array=w698) -> (element #1=w702:string, element #2=w694:string)  [unwired: 2 in]
                        n235 = Equal?(x="ON", y=w702) -> (x = y?=w701:bool)
                        n236 = Fract/Exp String To Number(string=w694) -> (number=w693:dbl)  [unwired: 3 in, 1 out]
                        n237 = Bundle By Name(cluster=w695, "Command"=w697, "SI camera info.Quartz"=w701, "SI camera info.Quartz Percent"=w693) -> (w705:T2)
                        n238 = Enqueue Element(queue=w700, element=w705, error in (no error)=w699) -> (error out=w704:errorcluster)  [unwired: 1 in, 2 out]
                        n239 = case shown="Error" w704 {
                          selector: w704 -> [w706 _]
                          tunnel: w696 -> [w708 w711]
                          tunnel: [w707 w710] -> w688
                          frame No Error {
                            n240 = call "TCP Write with Size.vi"("error in (no error)"=w706, "data in"="OK", "connection ID"=w708) -> ("error out"=w707:errorcluster)  [unwired: 6 in, 2 out]
                          }
                          frame Error {
                            n241 = call "TCP Write with Size.vi"("data in"="ERROR", "connection ID"=w711) -> ("error out"=w710:errorcluster)  [unwired: 7 in, 2 out]
                          }
                        }
                        n242 = Concatenate Strings(w691, "\r\n", w690) -> (w689:string)
                      }
                      frame "Fe" {
                        n243 = Index Array(array=w721) -> (element=w725:string)  [unwired: 1 in]
                        n244 = Equal?(x="ON", y=w725) -> (x = y?=w724:bool)
                        n245 = Bundle By Name(cluster=w718, "Command"=w720, "SI camera info.Fe"=w724) -> (w728:T2)
                        n246 = Enqueue Element(queue=w722, element=w728, error in (no error)=w723) -> (error out=w727:errorcluster)  [unwired: 1 in, 2 out]
                        n247 = case shown="Error" w727 {
                          selector: w727 -> [w729 _]
                          tunnel: w719 -> [w731 w734]
                          tunnel: [w730 w733] -> w717
                          frame No Error {
                            n248 = call "TCP Write with Size.vi"("error in (no error)"=w729, "data in"="OK", "connection ID"=w731) -> ("error out"=w730:errorcluster)  [unwired: 6 in, 2 out]
                          }
                          frame Error {
                            n249 = call "TCP Write with Size.vi"("data in"="ERROR", "connection ID"=w734) -> ("error out"=w733:errorcluster)  [unwired: 7 in, 2 out]
                          }
                        }
                        n250 = Concatenate Strings(w715, "\r\n", w714) -> (w713:string)
                      }
                      frame "LAMPS" {
                        n251 = Index Array(array=w766) -> (element #1=w757:string, element #2=w743:string, element #3=w756:string, element #4=w755:string, element #5=w754:string, element #6=w753:string, element #7=w742:string, element #8=w741:string, element #9=w737:string, element #10=w736:string)  [unwired: 10 in]
                        n252 = Bundle("String"=w757, "String"=w743, "String"=w756, "String"=w755, "String"=w754, "String"=w753, "String"=w742, "String"=w741) -> (w752:T11)  [unwired: 1 in]
                        n253 = Equal?(x="ON", y=w752) -> (x = y?=w751:T12)
                        n254 = Unbundle(w751) -> ("String"=w750:bool, "String"=w749:bool, "String"=w748:bool, "String"=w747:bool, "String"=w746:bool, "String"=w745:bool, "String"=w744:bool, "String"=w740:bool)
                        n255 = Fract/Exp String To Number(string=w737) -> (number=w739:dbl)  [unwired: 3 in, 1 out]
                        n256 = Fract/Exp String To Number(string=w736) -> (number=w738:dbl)  [unwired: 3 in, 1 out]
                        n257 = Bundle By Name(cluster=w763, "Command"=w765, "SI camera info.Hg(Ar)"=w750, "SI camera info.Cu"=w749, "SI camera info.Ne"=w748, "SI camera info.Bulb"=w747, "SI camera info.Ar"=w746, "SI camera info.Fe"=w745, "SI camera info.Quartz"=w744, "SI camera info.Dome"=w740, "SI camera info.Quartz Percent"=w739, "SI camera info.DomePercent"=w738) -> (w771:T2)
                        n258 = Enqueue Element(queue=w767, element=w771, error in (no error)=w768) -> (error out=w770:errorcluster)  [unwired: 1 in, 2 out]
                        n259 = case shown="Error" w770 {
                          selector: w770 -> [w772 _]
                          tunnel: w764 -> [w774 w777]
                          tunnel: [w773 w776] -> w762
                          frame No Error {
                            n260 = call "TCP Write with Size.vi"("error in (no error)"=w772, "data in"="OK", "connection ID"=w774) -> ("error out"=w773:errorcluster)  [unwired: 6 in, 2 out]
                          }
                          frame Error {
                            n261 = call "TCP Write with Size.vi"("data in"="ERROR", "connection ID"=w777) -> ("error out"=w776:errorcluster)  [unwired: 7 in, 2 out]
                          }
                        }
                        n262 = Concatenate Strings(w760, "\r\n", w759) -> (w758:string)
                      }
                      frame "SETUP" {
                        n263 = Index Array(array=w804) -> (element #1=w800:string, element #2=w781:string, element #3=w799:string, element #4=w798:string, element #5=w797:string, element #6=w795:string, element #7=w793:string, element #8=w791:string, element #9=w783:string, element #10=w788:string)  [unwired: 10 in]
                        n264 = Fract/Exp String To Number(string=w793) -> (number=w792:dbl)  [unwired: 3 in, 1 out]
                        n265 = Fract/Exp String To Number(string=w797) -> (number=w796:dbl)  [unwired: 3 in, 1 out]
                        n266 = Equal?(x=w783, y="TRUE") -> (x = y?=w789:bool)
                        n267 = Fract/Exp String To Number(string=w791) -> (number=w790:dbl)  [unwired: 3 in, 1 out]
                        n268 = Fract/Exp String To Number(string=w795) -> (number=w794:dbl)  [unwired: 3 in, 1 out]
                        n269 = local write "Setup Commanded"(TRUE) -> ()
                        n270 = local write "Setup Done"(FALSE) -> ()
                        n271 = Bundle By Name(cluster=w805, "Command"=w803, "Configuration.Primary Filter"=w800, "Configuration.Secondary Filter"=w781, "Configuration.Slit Mask"=w799, "Configuration.Grating"=w798, "Configuration.CS Target"=w796, "Configuration.GS Target"=w794, "Configuration.Camera Focus"=w792, "Configuration.Coll Focus"=w790, "Configuration.use Flexure Comp?"=w789, "Configuration.WavMode"=w788) -> (w809:T3)
                        n272 = Enqueue Element(queue=w802, element=w809, error in (no error)=w801) -> (error out=w808:errorcluster)  [unwired: 1 in, 2 out]
                        n273 = case shown="No Error" w808 {
                          selector: w808 -> [w810 _]
                          tunnel: w806 -> [w812 w815]
                          tunnel: [w811 w814] -> w807
                          frame No Error {
                            n274 = call "TCP Write with Size.vi"("error in (no error)"=w810, "data in"="OK", "connection ID"=w812) -> ("error out"=w811:errorcluster)  [unwired: 6 in, 2 out]
                          }
                          frame Error {
                            n275 = call "TCP Write with Size.vi"("data in"="ERROR", "connection ID"=w815) -> ("error out"=w814:errorcluster)  [unwired: 7 in, 2 out]
                          }
                        }
                        n276 = Concatenate Strings(w786, "\r\n", w785) -> (w784:string)
                      }
                      frame "FOCUS" {
                        n277 = Fract/Exp String To Number(string=w824) -> (number=w823:dbl[])  [unwired: 3 in, 1 out]
                        n278 = Index Array(array=w823) -> (element #1=w822:dbl, element #2=w821:dbl, element #3=w820:dbl)  [unwired: 3 in]
                        n279 = local write "Focus Done"(FALSE) -> ()
                        n280 = local write "Focus Commanded"(TRUE) -> ()
                        n281 = Bundle By Name(cluster=w825, "Command"=w831, "SI camera info.Start"=w822, "SI camera info.Delta"=w821, "SI camera info.Steps"=w820) -> (w835:T2)
                        n282 = Enqueue Element(queue=w819, element=w835, error in (no error)=w830) -> (error out=w834:errorcluster)  [unwired: 1 in, 2 out]
                        n283 = case shown="No Error" w834 {
                          selector: w834 -> [w836 _]
                          tunnel: w832 -> [w838 w841]
                          tunnel: [w837 w840] -> w833
                          frame No Error {
                            n284 = call "TCP Write with Size.vi"("error in (no error)"=w836, "data in"="OK", "connection ID"=w838) -> ("error out"=w837:errorcluster)  [unwired: 6 in, 2 out]
                          }
                          frame Error {
                            n285 = call "TCP Write with Size.vi"("data in"="ERROR", "connection ID"=w841) -> ("error out"=w840:errorcluster)  [unwired: 7 in, 2 out]
                          }
                        }
                        n286 = Concatenate Strings(w828, "\r\n", w827) -> (w826:string)
                      }
                      frame "CAMSET" {
                        n287 = Index Array(array=w871) -> (element #1=w872:string, element #2=w870:string, element #3=w869:string, element #4=w868:string, element #5=w844:string, element #6=w867:string, element #7=w866:string, element #8=w863:string, element #9=w853:string, element #10=w857:string, element #11=w848:string, element #12=w851:string, element #13=w850:string, element #14=w856:string, element #15=w849:string)  [unwired: 15 in]
                        n288 = Fract/Exp String To Number(string=w867) -> (number=w865:dbl)  [unwired: 3 in, 1 out]
                        n289 = Fract/Exp String To Number(string=w866) -> (number=w864:dbl)  [unwired: 3 in, 1 out]
                        n290 = Fract/Exp String To Number(string=w863, default (0 dbl)=u8 0) -> (number=w855:u8)  [unwired: 2 in, 1 out]
                        n291 = Fract/Exp String To Number(string=w844) -> (number=w845:dbl)  [unwired: 3 in, 1 out]
                        n292 = Fract/Exp String To Number(string=w853, default (0 dbl)=u16 0) -> (number=w862:u16)  [unwired: 2 in, 1 out]
                        n293 = Bundle("String"=w857, "String"=w848, "String"=w851, "String"=w850, "String"=w856, "String"=w849) -> (w852:T9)  [unwired: 1 in]
                        n294 = Fract/Exp String To Number(string=w852) -> (number=w854:T10)  [unwired: 3 in, 1 out]
                        n295 = Bundle By Name(cluster=w877, "Command"=w875, "SI camera info.Observer Name"=w872, "SI camera info.object name"=w870, "SI camera info.File name base"=w869, "SI camera info.Notes"=w868, "SI camera info.Exp type tab"=w845, "SI camera info.Number of Exp"=w865, "SI camera info.Exp time"=w864, "SI camera info.CCD Readout Speed"=w855, "SI camera info.CCD ROI Mode"=w862, "SI camera info.Custom Roi"=w854) -> (w880:T2)
                        n296 = Concatenate Strings(w859, "\r\n", w858) -> (w860:string)
                        n297 = Enqueue Element(queue=w874, element=w880, error in (no error)=w873) -> (error out=w879:errorcluster)  [unwired: 1 in, 2 out]
                        n298 = case shown="No Error" w879 {
                          selector: w879 -> [w881 _]
                          tunnel: w876 -> [w883 w886]
                          tunnel: [w882 w885] -> w878
                          frame No Error {
                            n299 = call "TCP Write with Size.vi"("error in (no error)"=w881, "data in"="OK", "connection ID"=w883) -> ("error out"=w882:errorcluster)  [unwired: 6 in, 2 out]
                          }
                          frame Error {
                            n300 = call "TCP Write with Size.vi"("data in"="ERROR", "connection ID"=w886) -> ("error out"=w885:errorcluster)  [unwired: 7 in, 2 out]
                          }
                        }
                        n301 = local write "Camset Done"(FALSE) -> ()
                      }
                      frame "START" {
                        n302 = Bundle By Name(cluster=w889, "Command"=w892) -> (w894:T2)
                        n303 = Enqueue Element(queue=w891, element=w894) -> (error out=w893:errorcluster)  [unwired: 2 in, 2 out]
                        n304 = case shown="No Error" w893 {
                          selector: w893 -> [w899 _]
                          tunnel: w890 -> [w901 w904]
                          tunnel: [w900 w903] -> w888
                          frame No Error {
                            n305 = call "TCP Write with Size.vi"("error in (no error)"=w899, "data in"="OK", "connection ID"=w901) -> ("error out"=w900:errorcluster)  [unwired: 6 in, 2 out]
                          }
                          frame Error {
                            n306 = call "TCP Write with Size.vi"("data in"="ERROR", "connection ID"=w904) -> ("error out"=w903:errorcluster)  [unwired: 7 in, 2 out]
                          }
                        }
                        n307 = Concatenate Strings(w897, "\r\n", w896) -> (w895:string)
                      }
                      frame "ABORT" {
                        n308 = Bundle By Name(cluster=w907, "Command"=w910) -> (w912:T2)
                        n309 = Enqueue Element(queue=w909, element=w912) -> (error out=w911:errorcluster)  [unwired: 2 in, 2 out]
                        n310 = case shown="No Error" w911 {
                          selector: w911 -> [w917 _]
                          tunnel: w908 -> [w919 w922]
                          tunnel: [w918 w921] -> w906
                          frame No Error {
                            n311 = call "TCP Write with Size.vi"("error in (no error)"=w917, "data in"="OK", "connection ID"=w919) -> ("error out"=w918:errorcluster)  [unwired: 6 in, 2 out]
                          }
                          frame Error {
                            n312 = call "TCP Write with Size.vi"("data in"="ERROR", "connection ID"=w922) -> ("error out"=w921:errorcluster)  [unwired: 7 in, 2 out]
                          }
                        }
                        n313 = Concatenate Strings(w915, "\r\n", w914) -> (w913:string)
                      }
                      frame "MIRROR" {
                        n314 = Index Array(array=w925) -> (element=w924:string)  [unwired: 1 in]
                        n315 = Equal?(x=w924, y="IN") -> (x = y?=w926:bool)
                        n316 = Bundle By Name(cluster=w931, "Command"="CLM", "TCS.Comp Mirror"=w926) -> (w930:T1)
                        n317 = Enqueue Element(queue=w932, element=w930) -> (error out=w928:errorcluster)  [unwired: 2 in, 2 out]
                        n318 = case shown="No Error" w928 {
                          tunnel: w934 -> [w940 w943]
                          tunnel: [w939 w942] -> w933
                          frame No Error {
                            n319 = call "TCP Write with Size.vi"("data in"="OK", "connection ID"=w940) -> ("error out"=w939:errorcluster)  [unwired: 7 in, 2 out]
                          }
                          frame Error {
                            n320 = call "TCP Write with Size.vi"("data in"="ERROR", "connection ID"=w943) -> ("error out"=w942:errorcluster)  [unwired: 7 in, 2 out]
                          }
                        }
                        n321 = Concatenate Strings(w937, "\r\n", w936) -> (w935:string)
                      }
                      frame "TARGET" {
                        n322 = Index Array(array=w949) -> (element #1=w946:string, element #2=w945:string)  [unwired: 2 in]
                        n323 = Bundle By Name(cluster=w951, "Command"=w947, "TCS.RA"=w946, "TCS.DEC"=w945) -> (w950:T1)
                        n324 = Enqueue Element(queue=w952, element=w950) -> (error out=w948:errorcluster)  [unwired: 2 in, 2 out]
                        n325 = case shown="No Error" w948 {
                          tunnel: w954 -> [w960 w963]
                          tunnel: [w959 w962] -> w953
                          frame No Error {
                            n326 = call "TCP Write with Size.vi"("data in"="OK", "connection ID"=w960) -> ("error out"=w959:errorcluster)  [unwired: 7 in, 2 out]
                          }
                          frame Error {
                            n327 = call "TCP Write with Size.vi"("data in"="ERROR", "connection ID"=w963) -> ("error out"=w962:errorcluster)  [unwired: 7 in, 2 out]
                          }
                        }
                        n328 = Concatenate Strings(w957, "\r\n", w956) -> (w955:string)
                      }
                      frame "TEST" {
                        n329 = case shown="No Error" w965 {
                          selector: w965 -> [w972 _]
                          tunnel: w967 -> [w974 w977]
                          tunnel: [w973 w976] -> w966
                          frame No Error {
                            n330 = call "TCPWriteWithSize.vi"("error in (no error)"=w972, "Command String"="OK" ("data in"), "Connection In"=w974) -> ("error out"=w973:errorcluster)  [unwired: 7 in, 1 out]
                          }
                          frame Error {
                            n331 = call "TCP Write with Size.vi"("data in"="ERROR", "connection ID"=w977) -> ("error out"=w976:errorcluster)  [unwired: 7 in, 2 out]
                          }
                        }
                        n332 = Concatenate Strings(w970, "\r\n", w969) -> (w968:string)
                      }
                    }
                  }
                }
                "Command History" <- w61
              }
              frame Error {
                n333 = Unbundle By Name(w980) -> ("code"=w981:i32)
                n334 = case shown="56" w981 {
                  tunnel: w980 -> [w982 _]
                  tunnel: [w982 errorcluster {"status"=FALSE, "code"=0, "source"=""} ("error IO")] -> w979
                  frame 0, Default {
                  }
                  frame 56 {
                  }
                }
              }
            }
          }
          frame "DONE" {
            n335 = case shown="\"FOCUS\"" w986 {
              tunnel: w985 -> [w993 w994 w996 w998]
              tunnel: [w993 w994 w996 w998] -> w984
              frame "", Default {
              }
              frame "SETUP", "SETUPNOCHANGE" {
                n336 = local write "Setup Done"(TRUE) -> ()
              }
              frame "CAMSET" {
                n337 = local write "Camset Done"(TRUE) -> ()
              }
              frame "FOCUS" {
                n338 = local write "Focus Done"(TRUE) -> ()
              }
            }
            n339 = local read "Setup Commanded"() -> (w987:bool)
            n340 = Concatenate Strings("DONE", "\t", w986) -> (w989:string)
            n341 = case shown="True" w987 {
              tunnel: w992 -> [w1010 w1029]
              tunnel: w984 -> [w1009 w1028]
              tunnel: [w1008 w1027] -> w991
              tunnel: w989 -> [_ w1026]
              frame True {
                n342 = local read "Focus Commanded"() -> (w1000:bool)
                n343 = local read "Camset Done"() -> (w1006:bool)
                n344 = local read "Setup Done"() -> (w1004:bool)
                n345 = local read "Focus Done"() -> (w1003:bool)
                n346 = Not(x=w1000) -> (.not. x?=w1001:bool)
                n347 = Or(x=w1003, y=w1001) -> (x .or. y?=w1002:bool)
                n348 = Build Array(w1006, w1004, w1002) -> (w1005:bool[])
                n349 = And Array Elements(Boolean array=w1005) -> (logical AND=w1007:bool)
                n350 = case shown="True" w1007 {
                  tunnel: w1010 -> [_ w1025]
                  tunnel: w1009 -> [w1011 w1024]
                  tunnel: [w1011 w1021] -> w1008
                  frame False {
                    # "Not all done commands received"
                  }
                  frame True {
                    w1020 = FALSE
                    n351 = local write "Camset Done"(w1020) -> ()
                    n352 = local write "Focus Commanded"(w1020) -> ()
                    n353 = local write "Focus Done"(w1020) -> ()
                    n354 = local write "Setup Done"(w1020) -> ()
                    n355 = local write "Setup Commanded"(w1020) -> ()
                    n356 = Concatenate Strings("DONE", "\t", "SETUP") -> (w1017:string)
                    n357 = call "TCP Write with Size.vi"("error in (no error)"=w1024, "data in"=w1017, "connection ID"=w1025) -> ("error out"=w1022:errorcluster, "connection ID out"=w1023:refnum<k5>)  [unwired: 6 in, 1 out]
                    n358 = Concatenate Strings("DONE", "\t", "CAMSET") -> (w1016:string)
                    n359 = call "TCP Write with Size.vi"("error in (no error)"=w1022, "data in"=w1016, "connection ID"=w1023) -> ("error out"=w1021:errorcluster)  [unwired: 6 in, 2 out]
                  }
                }
              }
              frame False {
                n360 = call "TCP Write with Size.vi"("error in (no error)"=w1028, "data in"=w1026, "connection ID"=w1029) -> ("error out"=w1027:errorcluster)  [unwired: 6 in, 2 out]
              }
            }
          }
          frame "IMAGE" {
            n361 = Equal?(x=w1035, y="STARTED") -> (x = y?=w1033:bool)
            n362 = case shown="True" w1033 {
              selector: w1033 -> [w1038 w1051]
              tunnel: w1032 -> [w1041 w1048]
              tunnel: w1031 -> [w1040 w1047]
              tunnel: [w1039 w1046] -> w1030
              frame False {
                # "Imaging done, pass up to SQM, unlock commands"
                n363 = local write "Exposure Active?"(w1038) -> ()
                n364 = Concatenate Strings("STATUS", "\t", "IMAGINGDONE") -> (w1042:string)
                n365 = call "TCP Write with Size.vi"("error in (no error)"=w1040, "data in"=w1042, "connection ID"=w1041) -> ("error out"=w1039:errorcluster)  [unwired: 6 in, 2 out]
              }
              frame True {
                # "imaging started, exposure active. Lock out other commands"
                n366 = local write "Exposure Active?"(w1051) -> ()
                n367 = Concatenate Strings("STATUS", "\t", "IMAGING") -> (w1049:string)
                n368 = call "TCP Write with Size.vi"("error in (no error)"=w1047, "data in"=w1049, "connection ID"=w1048) -> ("error out"=w1046:errorcluster)  [unwired: 6 in, 2 out]
              }
            }
          }
          frame "ERROR" {
            n369 = Concatenate Strings("ERROR", w1053) -> (w1052:string)
            n370 = call "TCP Write with Size.vi"("error in (no error)"=w1056, "data in"=w1052, "connection ID"=w1057) -> ("error out"=w1055:errorcluster)  [unwired: 6 in, 2 out]
          }
          frame "", Default {
            n371 = local read "Shutdown?"() -> (w1059:bool)
            n372 = case shown="False" w1059 {
              tunnel: w1062 -> [w1065 w1085]
              tunnel: w1061 -> [w1063 w1084]
              tunnel: [w1064 w1082] -> w1060
              tunnel: w1058 -> [w1066 _]
              frame True {
                n373 = local read "SI Server"() -> (w1071:bool)
                n374 = local read "TCS Server"() -> (w1070:bool)
                n375 = local read "Config Server"() -> (w1069:bool)
                n376 = Build Array(w1071, w1070, w1069) -> (w1068:bool[])
                n377 = Or Array Elements(Boolean array=w1068) -> (logical OR=w1067:bool)
                n378 = case shown="False" w1067 {
                  tunnel: w1066 -> [w1077 _]
                  tunnel: w1065 -> [w1075 w1081]
                  tunnel: [w1074 w1081] -> w1064
                  tunnel: w1063 -> [w1072 _]
                  frame False {
                    # "All Off"
                    n379 = Concatenate Strings("DONE", "\t", "Shutdown") -> (w1079:string)
                    n380 = Enqueue Element(queue=w1072, element=T4 {"Command"="SHUTDOWN", "Parameter"=""}) -> ()  [unwired: 2 in, 3 out]
                    n381 = call "TCP Write with Size.vi"("error in (no error)"=w1075, "data in"=w1079, "connection ID"=w1077) -> ("error out"=w1074:errorcluster)  [unwired: 6 in, 2 out]
                  }
                  frame True {
                    # "Still Waiting"
                  }
                }
              }
              frame False, Default {
                n382 = event shown="[0] Timeout" {
                  selector: _ -> [_ _]
                  dyn-events: _ -> [_ _]
                  timeout: 50 -> [_ _]
                  tunnel: w1085 -> [w1088 w1092]
                  tunnel: w1084 -> [w1089 w1093]
                  tunnel: [w1087 w1091] -> w1082
                  event Timeout {
                    n383 = event-data() -> ()  [unwired: 1 in, 2 out]
                    n384 = Enqueue Element(queue=w1089, element=T4 {"Command"="POLL", "Parameter"=""}, error in (no error)=w1088) -> (error out=w1087:errorcluster)  [unwired: 1 in, 2 out]
                  }
                  event Panel Close? {
                    n385 = event-data() -> ()  [unwired: 1 in, 4 out]
                    n386 = Enqueue Element(queue=w1093, element=T4 {"Command"="QUIT", "Parameter"=""}, error in (no error)=w1092) -> (error out=w1091:errorcluster)  [unwired: 1 in, 2 out]
                    n387 = event-data("Discard?"=TRUE) -> ()  [unwired: 1 in, 1 out]
                  }
                }
              }
            }
          }
          frame "QUIT" {
            n388 = case shown="\"TCS\"" w1095 {
              frame "", Default {
              }
              frame "TCS" {
                n389 = local write "TCS Server"(FALSE) -> ()
              }
              frame "SI" {
                n390 = local write "SI Server"(FALSE) -> ()
              }
              frame "CONFIG" {
                n391 = local write "Config Server"(FALSE) -> ()
              }
            }
          }
          frame "ACTIVE" {
            n392 = case shown="\"SI\"" w1100 {
              frame "", Default {
              }
              frame "TCS" {
                n393 = local write "TCS Server"(TRUE) -> ()
              }
              frame "SI" {
                n394 = local write "SI Server"(TRUE) -> ()
              }
              frame "CONFIG" {
                n395 = local write "Config Server"(TRUE) -> ()
              }
            }
          }
          frame "SHUTDOWN" {
            n396 = TCP Close Connection(connection ID=w1105) -> ()  [unwired: 2 in, 2 out]
          }
          frame "INIT" {
            w1108 = FALSE
            w1117 = 3
            w1119 = FALSE
            w1118 = FALSE
            # "and tcs server"
            # "open si & config servers"
            n397 = Current VI's Path() -> (path=w1138:path)
            n398 = Strip Path(path=w1138) -> (stripped path=w1130:path)  [unwired: 1 out]
            n399 = Strip Path(path=w1130) -> (stripped path=w1120:path)  [unwired: 1 out]
            n400 = Build Path(base path=w1120, name or relative path="Utils\\ChangeConfigServer.vi") -> (appended path=w1132:path)
            n401 = Build Path(base path=w1120, name or relative path="Utils\\ChangeSIServer.vi") -> (appended path=w1131:path)
            n402 = Build Path(base path=w1120, name or relative path="Utils\\ChangeTCSServer.vi") -> (appended path=w1122:path)
            n403 = local write "Config Server"(w1118) -> ()
            n404 = local write "TCS Server"(w1118) -> ()
            n405 = local write "SI Server"(w1118) -> ()
            n406 = Open VI Reference(vi path=w1132, error in (no error)=w1129) -> (vi reference=w1110:refnum<vi>)  [unwired: 4 in, 1 out]
            n407 = Open VI Reference(vi path=w1131, error in (no error)=w1129) -> (vi reference=w1114:refnum<vi>, error out=w1111:errorcluster)  [unwired: 4 in]
            n408 = Open VI Reference(vi path=w1122) -> (vi reference=w1116:refnum<vi>)  [unwired: 5 in, 1 out]
            n409 = local write "Command History"("") -> ()
            n410 = local write "Exposure Active?"(w1118) -> ()
            n411 = invoke class="VI" method="FP.Open"(reference=w1110, "State"=w1117) -> (reference out=w1109:refnum<vi>)  [unwired: 3 in, 4 out]
            n412 = invoke class="VI" method="FP.Open"(reference=w1114, error in=w1111, "State"=w1117) -> (reference out=w1113:refnum<vi>, error out=w1112:errorcluster)  [unwired: 2 in, 3 out]
            n413 = invoke class="VI" method="FP.Open"(reference=w1116, "State"=w1117) -> (reference out=w1115:refnum<vi>)  [unwired: 3 in, 4 out]
            n414 = local write "Shutdown?"(w1119) -> ()
            n415 = global write "TCP_Global.vi" "Shutdown"(w1119) -> ()
            n416 = invoke class="VI" method="Run VI"(reference=w1109, "Wait until done"=FALSE) -> (reference out=w1135:refnum<vi>, error out=w1127:errorcluster)  [unwired: 3 in, 3 out]
            n417 = invoke class="VI" method="Run VI"(reference=w1113, error in=w1112, "Wait until done"=FALSE) -> (reference out=w1133:refnum<vi>, error out=w1128:errorcluster)  [unwired: 2 in, 3 out]
            n418 = invoke class="VI" method="Run VI"(reference=w1115, "Wait until done"=FALSE) -> (reference out=w1123:refnum<vi>, error out=w1121:errorcluster)  [unwired: 3 in, 3 out]
            n419 = Close Reference(reference=w1135, error in (no error)=w1127) -> ()  [unwired: 1 out]
            n420 = Close Reference(reference=w1133, error in (no error)=w1128) -> (error out=w1126:errorcluster)
            n421 = Close Reference(reference=w1123, error in (no error)=w1121) -> ()  [unwired: 1 out]
            n422 = local write "Camset Done"(w1108) -> ()
            n423 = local write "Focus Commanded"(w1108) -> ()
            n424 = local write "Focus Done"(w1108) -> ()
            n425 = local write "Setup Done"(w1108) -> ()
            n426 = local write "Setup Commanded"(w1108) -> ()
          }
        }
      }
    }
    frame Error {
    }
  }
  "error out" <- w11
